vi "Obtain Credito from Dinero.vi"(8 "error in (no error)":errorcluster, 10 "Credito":i32, 11 "UI in":refnum<class "UI.lvclass">) -> (0 "error out":errorcluster, 3 "UI out":refnum<class "UI.lvclass">)   [LabVIEW 2020, in "UI.lvlib" / "UI.lvclass"]
uses:
  UI.lvclass
  UI.lvclass/UI.ctl
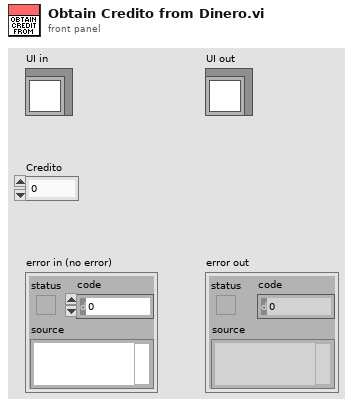
[diagram p1: front panel]
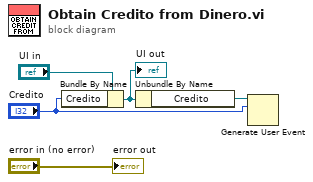
[diagram p0: block diagram]
diagram:
  n1 = Bundle By Name(cluster="UI in", "Credito"="Credito") -> (w2:refnum<class "UI.lvclass">)
  "UI out" <- w2
  n2 = Unbundle By Name(w2) -> ("Credito"=w1:refnum<user-event>)
  n3 = Generate User Event(user event=w1, event data cluster="Credito") -> ()  [unwired: 2 in, 2 out]
  "error out" <- "error in (no error)"
